vi "DigitalIO_ChannelLookup_Test.vi"() -> ()   [LabVIEW 2021]
uses:
  labbCAN_Bus_API/labbCAN_Bus_API.lvlib
  labbCAN_DigIO_API/labbCAN_DigIO_API.lvlib
panel:
  out "Digital In Channels":string[](array[string])
  out "Digital Out Channels":string[](array[string])
  out "Input Channel Count":i32
  out "Output Channel Count":i32
  out "error out":errorcluster caption="Fehler (Ausgang)"
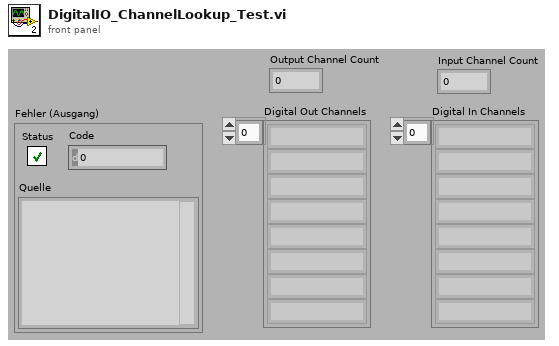
[diagram p1: front panel]
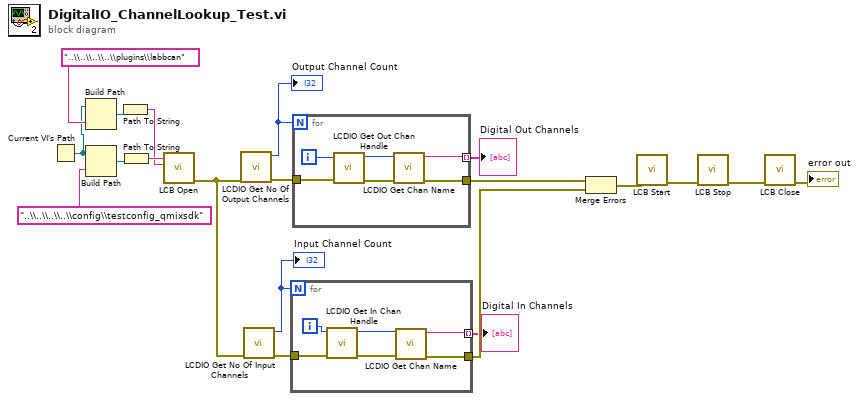
[diagram p0: block diagram]
diagram:
  n1 = Current VI's Path() -> (path=w12:path)
  n2 = Build Path(base path=w12, name or relative path="..\\..\\..\\..\\plugins\\labbcan" ("Name oder relativer Pfad")) -> (appended path=w14:path)
  n3 = Build Path(base path=w12, name or relative path="..\\..\\..\\..\\config\\testconfig_qmixsdk" ("Name oder relativer Pfad")) -> (appended path=w16:path)
  n4 = Path To String(path=w14) -> (string=w11:string)
  n5 = Path To String(path=w16) -> (string=w19:string)
  n6 = call "LCB Open.vi"("PluginSearchPath"=w11, "Device Configuration Path"=w19) -> ("error out"=w7:errorcluster)  [unwired: 9 in]
  n7 = call "LCDIO Get No Of Output Channels.vi"("error in (no error)"=w7) -> ("error out"=w8:errorcluster, "Output Channel Count"=w9:i32)  [unwired: 9 in]
  "Output Channel Count" <- w9
  n8 = call "LCDIO Get No Of Input Channels.vi"("error in (no error)"=w7) -> ("error out"=w6:errorcluster, "Input Channel Count"=w5:i32)  [unwired: 9 in]
  "Input Channel Count" <- w5
  n9 = for {
    N: w5 -> [_]
    tunnel: w6 -> [w25]
    tunnel: [w22] -> w3
    tunnel: [w21] -> w1 mode=indexing
    i -> [w26]
    n10 = call "LCDIO Get In Chan Handle.vi"("error in (no error)"=w25, "Index"=w26) -> ("error out"=w24:errorcluster, "Digital Input Channel"=w23:i64)  [unwired: 8 in]
    n11 = call "LCDIO Get Chan Name.vi"("error in (no error)"=w24, "Channel Handle"=w23) -> ("error out"=w22:errorcluster, "Name"=w21:string)  [unwired: 8 in]
  }
  "Digital In Channels" <- w1
  n12 = for {
    N: w9 -> [_]
    tunnel: w8 -> [w31]
    tunnel: [w28] -> w4
    tunnel: [w27] -> w2 mode=indexing
    i -> [w32]
    n13 = call "LCDIO Get Out Chan Handle.vi"("error in (no error)"=w31, "Index"=w32) -> ("error out"=w30:errorcluster, "Digital Output Channel"=w29:i64)  [unwired: 8 in]
    n14 = call "LCDIO Get Chan Name.vi"("error in (no error)"=w30, "Channel Handle"=w29) -> ("error out"=w28:errorcluster, "Name"=w27:string)  [unwired: 8 in]
  }
  "Digital Out Channels" <- w2
  n15 = Merge Errors(w4, w3) -> (w10:errorcluster)
  n16 = call "LCB Start.vi"("error in (no error)"=w10) -> ("error out"=w15:errorcluster)  [unwired: 10 in]
  n17 = call "LCB Stop.vi"("error in (no error)"=w15) -> ("error out"=w18:errorcluster)  [unwired: 10 in]
  n18 = call "LCB Close.vi"("error in (no error)"=w18) -> ("error out"=→"error out":errorcluster)  [unwired: 10 in]
